vi "Build Feed for Offline Installer.vi"(8 "error in":errorcluster, 10 "package name":string, 11 "OutputDir":path=path "C:/LUGE_2024.2/Demonstration/Builds/Offline Sources") -> (0 "error out":errorcluster)   [LabVIEW 2022 SP3, in "NIPM_Functions.lvlib"]
uses:
  NIPM_Functions.lvlib
  <vilib>/National Instruments/NIPM API (Beta)/NIPM_API.lvlib
panel:
  out "feed created?":bool
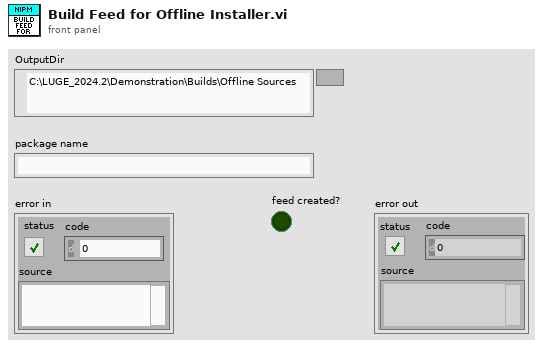
[diagram p1: front panel]
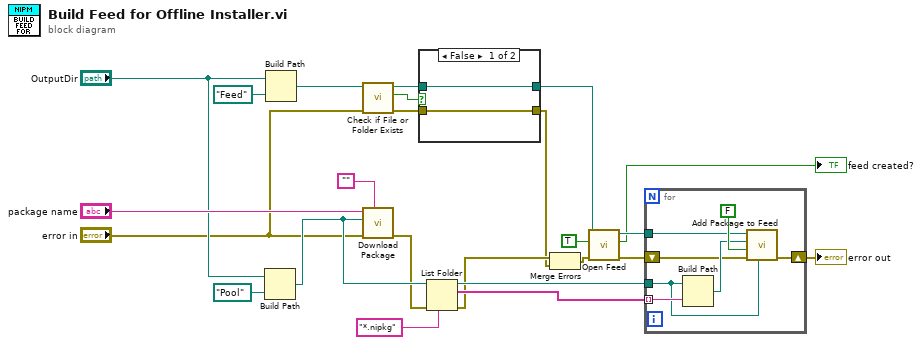
[diagram p0: block diagram]
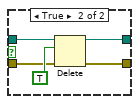
[diagram p2: hidden frame]
diagram:
  n1 = Build Path(base path="OutputDir", name or relative path=path "Pool") -> (appended path=w22:path)
  n2 = Build Path(base path="OutputDir", name or relative path=path "Feed") -> (appended path=w21:path)
  n3 = call <vilib>:"Check if File or Folder Exists.vi"("error in (no error)"="error in", "path"=w21) -> ("error out"=w13:errorcluster, "file or folder exists?"=w14:bool, "dup path"=w15:path)  [unwired: 7 in]
  n4 = call <vilib>:"Download Package.vi"("version (latest)"="", "error in"="error in", "destination folder"=w22, "package name"="package name") -> ("error out"=w11:errorcluster)  [unwired: 7 in]
  n5 = case shown="False" w14 {
    tunnel: w15 -> [w26 w30]
    tunnel: w13 -> [w25 w29]
    tunnel: [w25 w28] -> w7
    tunnel: [w26 w27] -> w9
    frame False {
    }
    frame True {
      n6 = Delete(path (use dialog)=w30, entire hierarchy (F)=TRUE, error in=w29) -> (deleted path=w27:path, error out=w28:errorcluster)  [unwired: 2 in, 1 out]
    }
  }
  n7 = List Folder(path=w22, pattern="*.nipkg", error in=w11) -> (path out=w16:path, filenames=w18:string[], error out=w10:errorcluster)  [unwired: 1 in, 1 out]
  n8 = Merge Errors(w10, w7) -> (w8:errorcluster)
  n9 = call <vilib>:"Open Feed.vi"("error in"=w8, "create feed if necessary (F)"=TRUE, "feed folderpath"=w9) -> ("error out"=w12:errorcluster, "feed created?"=→"feed created?":bool, "feed folderpath out"=w20:path)  [unwired: 6 in]
  n10 = for {
    tunnel: w20 -> [w36]
    tunnel: w18 -> [w38] mode=indexing
    tunnel: w16 -> [w34]
    shift-right: [w32] -> w2
    shift-left: w12 -> [w33]
    n11 = Build Path(base path=w34, name or relative path=w38) -> (appended path=w35:path)
    n12 = call <vilib>:"Add Package to Feed.vi"("package destination folderpath"=w34, "error in"=w33, "overwrite existing package (T)"=FALSE, "package source filepath"=w35, "feed folderpath in"=w36) -> ("error out"=w32:errorcluster)  [unwired: 4 in, 2 out]
  }
  "error out" <- w2
